vi "Tipo de guardado.vi"(8 "error in (no error)":errorcluster, 10 "Tipo de Guardado":enum16{"Tdms", "Txt"}(ring), 11 "Generador de Funciones in":refnum<class "Generador de Funciones.lvclass">) -> (0 "error out":errorcluster, 3 "Generador de Funciones out":refnum<class "Generador de Funciones.lvclass">)   [LabVIEW 2020, in "Generador de Funciones.lvlib" / "Generador de Funciones.lvclass"]
uses:
  Generador de Funciones.lvclass
  C:/Program Files (x86)/National Instruments/LabVIEW 2020/vi.lib/ActorFramework/Actor/Actor.lvclass
  Generador de Funciones.lvclass/Generador de Funciones.ctl
  Logging Tdms/Logging Tdms/Logging Tdms.lvclass
  C:/Users/Alex/Documents/Tarea-Actor/Logging Txt/Logging Txt/Logging Txt.lvclass
  Logging Txt/Logging Txt/Logging Txt.lvclass
  <vilib>/ActorFramework/Message Enqueuer/Message Enqueuer.lvclass/Message Enqueuer.ctl
  <vilib>/ActorFramework/Message Enqueuer/Enqueue.vi
  <vilib>/ActorFramework/Stop Msg/Stop Msg.lvclass
  C:/Program Files (x86)/National Instruments/LabVIEW 2020/vi.lib/ActorFramework/Message/Message.lvclass
  <vilib>/ActorFramework/Message Priority Queue/Priority Enqueue.vi
  <vilib>/ActorFramework/Actor/Actor.lvclass
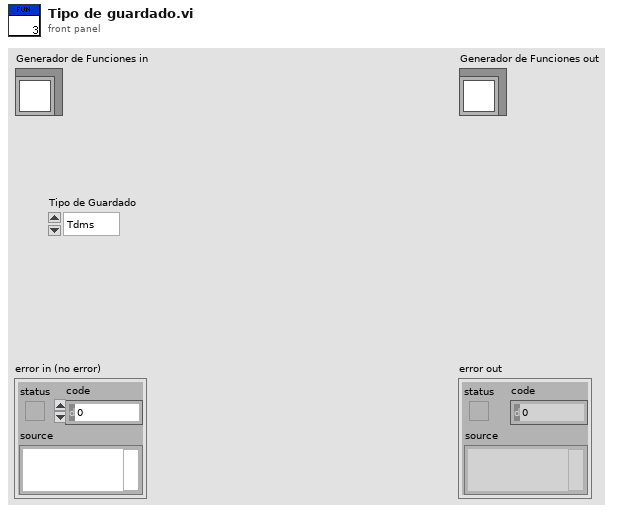
[diagram p1: front panel]
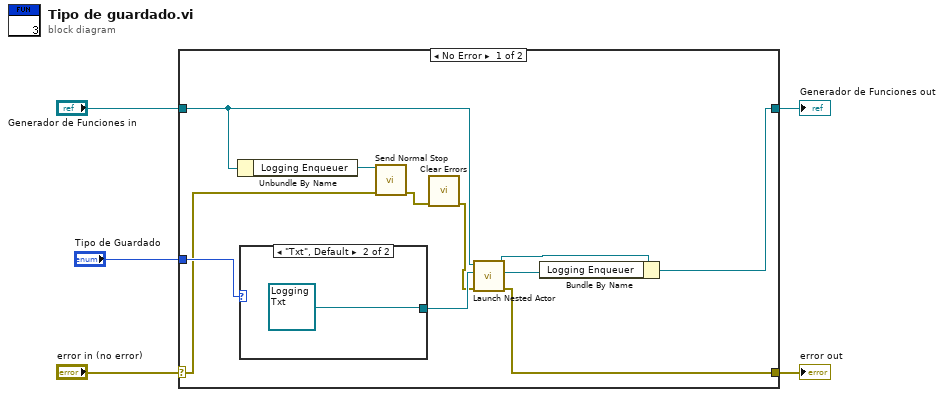
[diagram p0: block diagram]
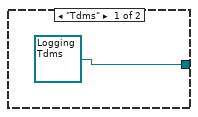
[diagram p2: hidden frame]
diagram:
  n1 = case shown="No Error" "error in (no error)" {
    selector: "error in (no error)" -> [w7 w20]
    tunnel: [w6 w20] -> w4
    tunnel: [w12 w19] -> w2
    tunnel: "Generador de Funciones in" -> [w15 w19]
    tunnel: "Tipo de Guardado" -> [w16 _]
    frame No Error {
      n2 = Unbundle By Name(w15) -> ("Logging Enqueuer"=w10:refnum<class "Message Enqueuer.lvclass">)
      n3 = case shown="\"Txt\", Default" w16 {
        tunnel: [refnum<class "Logging Tdms.lvclass"> refnum ("Logging Tdms.lvlib:Logging Tdms.lvclass") refnum<class "Logging Txt.lvclass"> refnum ("Logging Txt.lvlib:Logging Txt.lvclass")] -> w14
        frame "Tdms" {
        }
        frame "Txt", Default {
        }
      }
      n4 = call <vilib>:"Send Normal Stop.vi"("error in (no error)"=w7, "Message Enqueuer"=w10) -> ("error out"=w9:errorcluster)  [unwired: 9 in]
      n5 = call <vilib>:"Clear Errors.vi"("error in (no error)"=w9) -> ("error out"=w8:errorcluster)  [unwired: 5 in, 1 out]
      n6 = call <vilib>:"Launch Nested Actor.vi"("error in (no error)"=w8, "Nested Actor"=w14, "Caller Actor in"=w15) -> ("error out"=w6:errorcluster, "Nested Actor's Enqueuer"=w11:refnum<class "Message Enqueuer.lvclass">, "Caller Actor out"=w13:refnum<class "Generador de Funciones.lvclass">)  [unwired: 6 in]
      n7 = Bundle By Name(cluster=w13, "Logging Enqueuer"=w11) -> (w12:refnum<class "Generador de Funciones.lvclass">)
    }
    frame Error {
    }
  }
  "error out" <- w4
  "Generador de Funciones out" <- w2
